vi "manual close and deinit.vi"() -> ()   [LabVIEW 2021]
panel:
  out "return type 2":i16
  out "return value":i16
  out "error out":errorcluster
  in  "error in (no error)":errorcluster
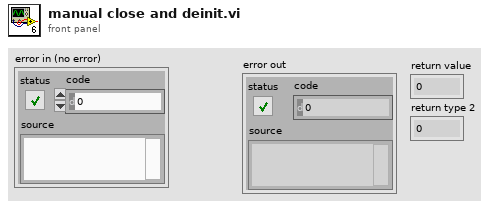
[diagram p1: front panel]
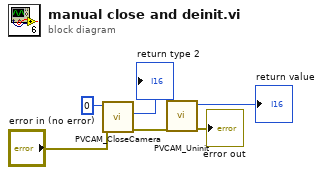
[diagram p0: block diagram]
diagram:
  n1 = call "PVCAM_CloseCamera.vi"("error in (no error)"="error in (no error)", "hCam"=i16 0) -> ("error out"=w4:errorcluster, "return type 2"=→"return type 2":i16)  [unwired: 8 in]
  n2 = call "PVCAM_Uninit.vi"("error in (no error)"=w4) -> ("error out"=→"error out":errorcluster, "return value"=→"return value":i16)  [unwired: 9 in]
